vi "Publisher.vi"() -> ()   [LabVIEW 2015]
doc: "The myRIO Project template acquires acceleration data from the onboard accelerometer and displays the changes of acceleration values in a waveform chart."
uses:
  <vilib>/daq.io/MQTT LabVIEW Client/Controls/QoS.ctl
  <vilib>/daq.io/MQTT LabVIEW Client/Controls/Retain_Flag.ctl
  <vilib>/daq.io/MQTT LabVIEW Client/Controls/DUP_Flag.ctl
  <vilib>/daq.io/MQTT LabVIEW Client/Controls/Connection_Return_Codes.ctl
  <vilib>/Instr/_visa.llb/VISA Configure Serial Port (Instr).vi
  <vilib>/daq.io/MQTT LabVIEW Client/MQTT_Functions.lvlib
panel:
  out "Stop All":bool
  in  "Stop Button":bool
  out "Publisher Connection Status":T1=enum."Connection refused: not authorized"
  in  "Message ID":u16=10
  in  "Publish Meta":cluster{"QoS":T2, "Retain":T3, "DUP":T4}
  in  "Topic":string="data"
  in  "MQTT Broker":cluster{"address (IP)":string, "port":u16}={"address (IP)"="52.37.169.179", "port"=1883}
  in  "Client ID":string="myRIO"
  out "CSV Output":string
  # "Connection Setup"
  # "DATA"
  # "Publish Set Up"
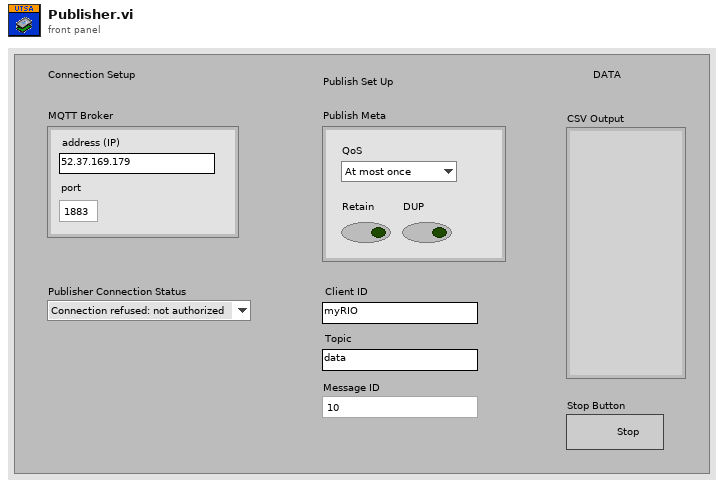
[diagram p1: front panel]
types:
  T1 = typedef "MQTT_Functions.lvlib/Connection_Return_Codes.ctl" = enum16{"Connection accepted", "Connection refused: unacceptable protocol version", "Connection refused: identifier rejected", "Connection refused: Server unavailable", "Connection refused: bad user name or password", "Connection refused: not authorized"}
  T2 = typedef "MQTT_Functions.lvlib/QoS.ctl" = enum8{"At most once", "At least once", "Exactly once", "Reserved"}
  T3 = typedef "MQTT_Functions.lvlib/Retain_Flag.ctl" = bool
  T4 = typedef "MQTT_Functions.lvlib/DUP_Flag.ctl" = bool
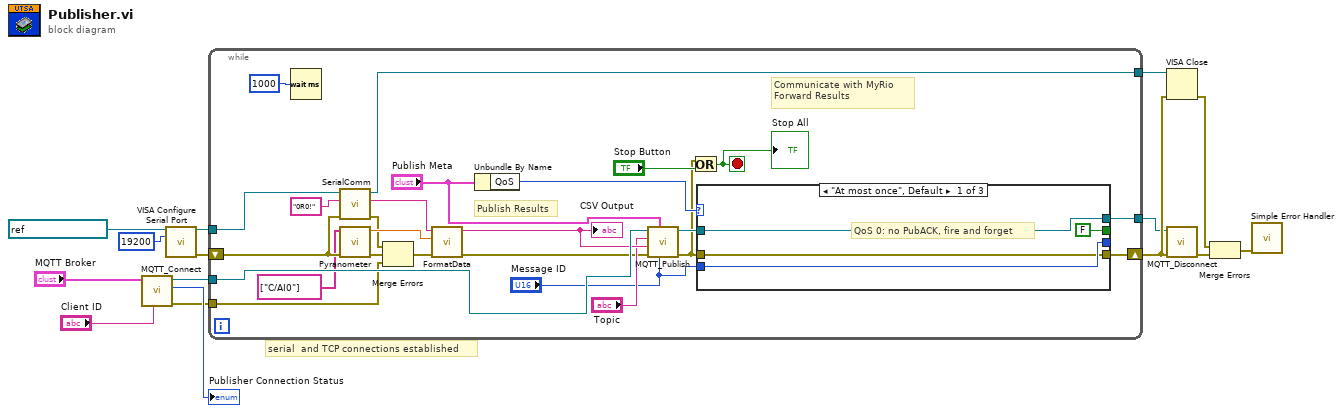
[diagram p0: block diagram]
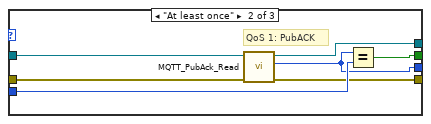
[diagram p2: hidden frame]
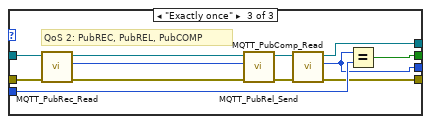
[diagram p3: hidden frame]
diagram:
  # "serial  and TCP connections established"
  n1 = call <vilib>:"MQTT_Connect.vi"("Client ID"="Client ID", "MQTT Broker"="MQTT Broker") -> ("error out"=w4:errorcluster, "Connection Status"=→"Publisher Connection Status":T1, "connection ID out"=w9:refnum<k5>)  [unwired: 7 in]
  n2 = call-poly "VISA Configure Serial Port"("VISA resource name"=refnum<visa-resource-name> "ASRL1::INSTR", "baud rate (9600)"=u32 19200) -> ("VISA resource name out"=w15:refnum<visa-resource-name>, "error out"=w14:errorcluster)  [unwired: 12 in]
  n3 = while {
    tunnel: w9 -> [w37]
    tunnel: w4 -> [w27]
    shift-right: [w17] -> w8
    shift-left: w14 -> [w39]
    tunnel: w15 -> [w40]
    tunnel: [w38] -> w11
    tunnel: [w16] -> w2
    stop <- w23 stop-if-true
    # "Publish Results"
    # "Communicate with MyRio\nForward Results"
    n4 = Wait (ms)(milliseconds to wait=u32 1000) -> ()  [unwired: 1 out]
    n5 = call "SerialComm.vi"("error in (no error)"=w39, "Write Command"="0R0!", "VISA Refnum in"=w40) -> ("error out"=w31:errorcluster, "Read Buffer"=w35:string, "VISA Refnum out"=w38:refnum<visa-resource-name>)  [unwired: 6 in]
    n6 = call "Pyranometer.vi"("error in (no error)"=w39, "Channel Names"=tag[] ["C/AI0"]) -> ("error out"=w32:errorcluster, "Output"=w34:dbl)  [unwired: 8 in]
    n7 = Merge Errors(w31, w32, w27) -> (w30:errorcluster)
    n8 = call "FormatData.vi"("error in (no error)"=w30, "Irradiance"=w34, "Read Buffer"=w35) -> ("error out"=w25:errorcluster, "CSV Output"=w29:string)  [unwired: 7 in]
    "CSV Output" <- w29
    n9 = Unbundle By Name("Publish Meta") -> ("QoS"=w22:T2)
    n10 = call <vilib>:"MQTT_Publish.vi"("Message ID"="Message ID", "Publish Meta"="Publish Meta", "error in (no error)"=w25, "Message to be published"=w29, "Topic"="Topic", "connection ID"=w37) -> ("error out"=w19:errorcluster, "connection ID out"=w20:refnum<k5>)  [unwired: 4 in]
    n11 = Or(x=w19, y="Stop Button") -> (x .or. y?=w23:bool)
    "Stop All" <- w23
    n12 = case shown="\"At most once\", Default" w22 {
      tunnel: w20 -> [w44 w51 w63]
      tunnel: [w41 w49 w56] -> w17
      tunnel: [w44 w48 w57] -> w16
      tunnel: "Message ID" -> [w42 w50 w62]
      tunnel: [FALSE w47 w58] -> _
      tunnel: [w42 w46 w55] -> _
      tunnel: w19 -> [w41 w45 w52]
      frame "At most once", Default {
        # "QoS 0: no PubACK, fire and forget"
      }
      frame "At least once" {
        # "QoS 1: PubACK"
        n13 = call <vilib>:"MQTT_PubAck_Read.vi"("error in (no error)"=w45, "connection ID"=w51) -> ("error out"=w49:errorcluster, "Message ID"=w46:u16, "connection ID out"=w48:refnum<k5>)  [unwired: 7 in]
        n14 = Equal?(x=w46, y=w50) -> (x = y?=w47:bool)
      }
      frame "Exactly once" {
        # "QoS 2: PubREC, PubREL, PubCOMP"
        n15 = call <vilib>:"MQTT_PubRec_Read.vi"("error in (no error)"=w52, "connection ID"=w63) -> ("error out"=w61:errorcluster, "Message ID"=w59:u16, "connection ID out"=w60:refnum<k5>)  [unwired: 7 in]
        n16 = call <vilib>:"MQTT_PubRel_Send.vi"("error in (no error)"=w61, "Message ID"=w59, "connection ID"=w60) -> ("error out"=w53:errorcluster, "connection ID out"=w54:refnum<k5>)  [unwired: 6 in, 1 out]
        n17 = call <vilib>:"MQTT_PubComp_Read.vi"("error in (no error)"=w53, "connection ID"=w54) -> ("error out"=w56:errorcluster, "Message ID"=w55:u16, "connection ID out"=w57:refnum<k5>)  [unwired: 7 in]
        n18 = Equal?(x=w55, y=w62) -> (x = y?=w58:bool)
      }
    }
  }
  n19 = VISA Close(VISA resource name=w11, error in (no error)=w8) -> (error out=w3:errorcluster)
  n20 = call <vilib>:"MQTT_Disconnect.vi"("error in (no error)"=w8, "connection ID"=w2) -> ("error out"=w7:errorcluster)  [unwired: 9 in]
  n21 = Merge Errors(w3, w7) -> (w6:errorcluster)
  n22 = call <vilib>:"Simple Error Handler.vi"("error in (no error)"=w6) -> ()  [unwired: 4 in, 5 out]
